vi "SPI Write Byte.vi"() -> ()   [LabVIEW 2023, in "CTI-Visa-Scratchpad.lvlib"]
uses:
  CTI-Visa-Scratchpad.lvlib
  CTI-Visa/CTI-Visa.lvlib
  CTI-Visa/SPI Config.ctl
panel:
  out "error out":errorcluster
  in  "Baud":u32=500000 format="%.0p"
  in  "Bus":u8
  in  "SPI Config":T1={"Mode"=0, "Data Bits"=8, "MOSI Pin"=7, "MISO Pin"=4, "SCK Pin"=6}
  in  "Port":refnum<visa-resource-name>="COM4"
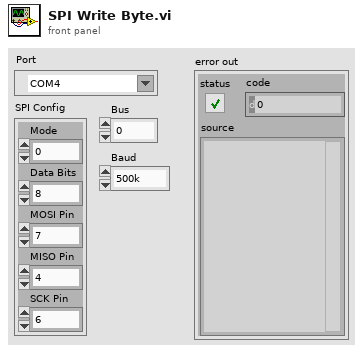
[diagram p1: front panel]
types:
  T1 = typedef "CTI-Visa.lvlib/SPI Config.ctl" = cluster{"Mode":u8, "Data Bits":u8, "MOSI Pin":u8, "MISO Pin":u8, "SCK Pin":u8}
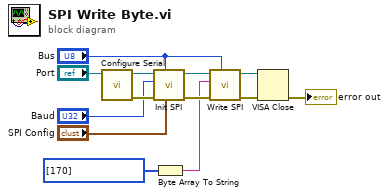
[diagram p0: block diagram]
diagram:
  n1 = call "Configure Serial.vi"("VISA resource name in"="Port") -> ("error out"=w12:errorcluster, "VISA resource name"=w11:refnum<visa-resource-name>)  [unwired: 9 in]
  n2 = call "Init SPI.vi"("SPI Config"="SPI Config", "Bus"="Bus", "error in (no error)"=w12, "Baud"="Baud", "VISA resource name in"=w11) -> ("error out"=w9:errorcluster, "VISA resource name"=w10:refnum<visa-resource-name>)  [unwired: 5 in]
  n3 = Byte Array To String(unsigned byte array=u8[] [170]) -> (string=w3:string)
  n4 = call "Write SPI.vi"("Bus"="Bus", "error in (no error)"=w9, "Data"=w3, "VISA resource name in"=w10) -> ("error out"=w7:errorcluster, "VISA resource name"=w6:refnum<visa-resource-name>)  [unwired: 6 in]
  n5 = VISA Close(VISA resource name=w6, error in (no error)=w7) -> (error out=→"error out":errorcluster)
